vi "Query All Channels.vi"(6 "timeout (ms)":i32=5000, 8 "error in":errorcluster, 10 "Channel Filter":T4, 11 "gRPC ID in":T6) -> (0 "error out":errorcluster, 2 "channels":T1[](array[typedef]), 3 "gRPC ID out":T6)   [LabVIEW 2021, in "CIFManagerClientWrapper.lvlib"]
uses:
  CIFManagerClientWrapper.lvlib
  <vilib>/gRPC/LabVIEW gRPC Library/Shared/grpcId.ctl
  CIF_Manager_client/RPC Messages/cif_manager_QueryAllChannelsRequest.ctl
  CIF_Manager_client/RPC Messages/cif_management_common_ChannelFilter.ctl
  CIF_Manager_client/RPC Messages/cif_management_common_ChannelDirection.ctl
  CIF_Manager_client/RPC Messages/cif_management_common_Channel.ctl
  CIF_Manager_client/RPC Messages/cif_management_common_ChannelPattern.ctl
  CIF_Manager_client/CIF_Manager_client.lvlib
  <vilib>/gRPC/LabVIEW gRPC Library/grpc-lvsupport-release.lvlib
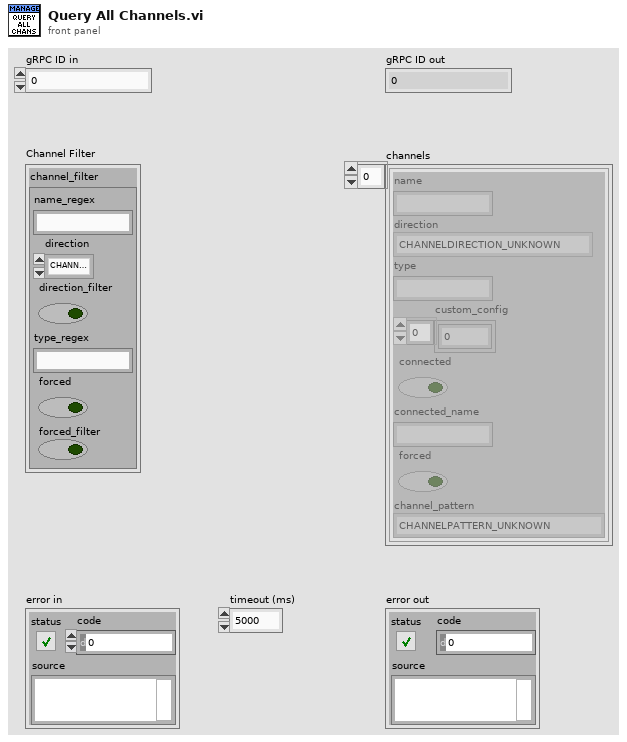
[diagram p1: front panel]
types:
  T1 = typedef "CIF_Manager_client.lvlib/cif_management_common_Channel.ctl" = cluster{"name":string, "direction":T2, "type":string, "custom_config":u8[], "connected":bool, "connected_name":string, "forced":bool, "channel_pattern":T3}
  T2 = typedef "CIF_Manager_client.lvlib/cif_management_common_ChannelDirection.ctl" = enum32{"CHANNELDIRECTION_UNKNOWN", "CHANNELDIRECTION_PUBLISHER", "CHANNELDIRECTION_SUBSCRIBER"}
  T3 = typedef "CIF_Manager_client.lvlib/cif_management_common_ChannelPattern.ctl" = enum32{"CHANNELPATTERN_UNKNOWN", "CHANNELPATTERN_TAG", "CHANNELPATTERN_FIFO", "CHANNELPATTERN_MULTIFIFO", "CHANNELPATTERN_BACKPRESSUREFIFO"}
  T4 = typedef "CIF_Manager_client.lvlib/cif_manager_QueryAllChannelsRequest.ctl" = cluster{"channel_filter":T5}
  T5 = typedef "CIF_Manager_client.lvlib/cif_management_common_ChannelFilter.ctl" = cluster{"name_regex":string, "direction":T2, "direction_filter":bool, "type_regex":string, "forced":bool, "forced_filter":bool}
  T6 = typedef "grpc-lvsupport-release.lvlib/grpcId.ctl" = u64
  T7 = typedef "CIF_Manager_client.lvlib/cif_manager_QueryAllChannelsResponse.ctl" = cluster{"channels":T8}
  T8 = typedef "CIF_Manager_client.lvlib/cif_management_common_Channels.ctl" = cluster{"channels":T1[]}
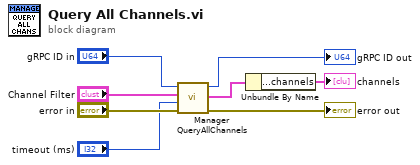
[diagram p0: block diagram]
diagram:
  n1 = call "Manager QueryAllChannels.vi"("error in"="error in", "timeout (ms)"="timeout (ms)", "Request Data"="Channel Filter", "gRPC ID"="gRPC ID in") -> ("error out"=→"error out":errorcluster, "Response Data"=w4:T7, "gRPC ID out"=→"gRPC ID out":T6)  [unwired: 5 in]
  n2 = Unbundle By Name(w4) -> ("channels.channels"=→"channels":T1[])
